vi "反馈节点.vi"() -> ()   [LabVIEW 2020]
doc: "本VI是为《我和LabVIEW》一书编写的示例。\n关于本书的介绍请参考网页：\nhttp://ruanqizhen.spaces.live.com/blog/cns!5852D4F797C53FB6!4310.entry"
panel:
  out "数值":i32
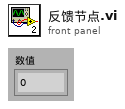
[diagram p1: front panel]
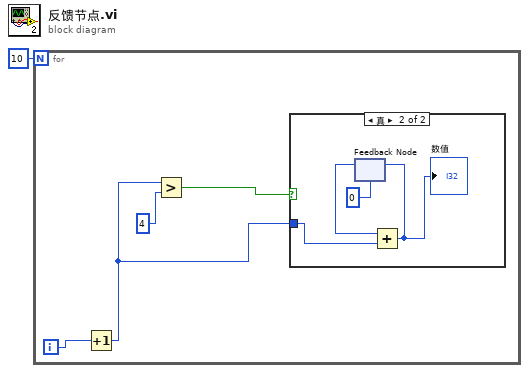
[diagram p0: block diagram]
diagram:
  n1 = for {
    N: 10 -> [_]
    i -> [w5]
    n2 = Increment(x=w5) -> (x+1=w2:i32)
    n3 = Greater?(x=w2, y=4) -> (0:w3:bool)
    n4 = case shown="真" w3 {
      tunnel: w2 -> [_ w9]
      frame False {
      }
      frame True {
        n5 = feedback #1(0) -> (w7:i32)
        n6 = Add(x=w7, y=w9) -> (x+y=w8:i32)
        "数值" <- w8
        n7 = feedback-in #1(w8) -> ()
      }
    }
  }
